vi "Engine 2 UI.vi"() -> ()   [LabVIEW 2015]
panel:
  out "Boolean_in":bool caption="Boolean"
  out "dbl_in":dbl caption="Double"
  out "String_in":string caption="String"
  out "U8_array_in":u8[](array[numeric]) caption="Array of U8"
  out "U8_in":u8 caption="U8"
  out "U16_in":u16 caption="U16"
  in  "Boolean_out":bool caption="Boolean"
  in  "dbl_out":dbl caption="Double"
  in  "String_out":string caption="String"
  in  "U8_array_out":u8[](array[numeric]) caption="Array of U8"
  in  "U8_out":u8 caption="U8"
  in  "U16_out":u16 caption="U16"
  out "Last Update":dbl format="%<%H:%M:%S>T"
  # "Input"
  # "Output"
  # "The UDP transfer mechanism allows the\nuser to configure a last update tag."
  # "Some data types are only compatible with\nspecific transfer mechanisms. For example:\nthe UDP transfer mechanism supports \nstrings and arrays, while the RT FIFO\ntransfer mechanism does not."
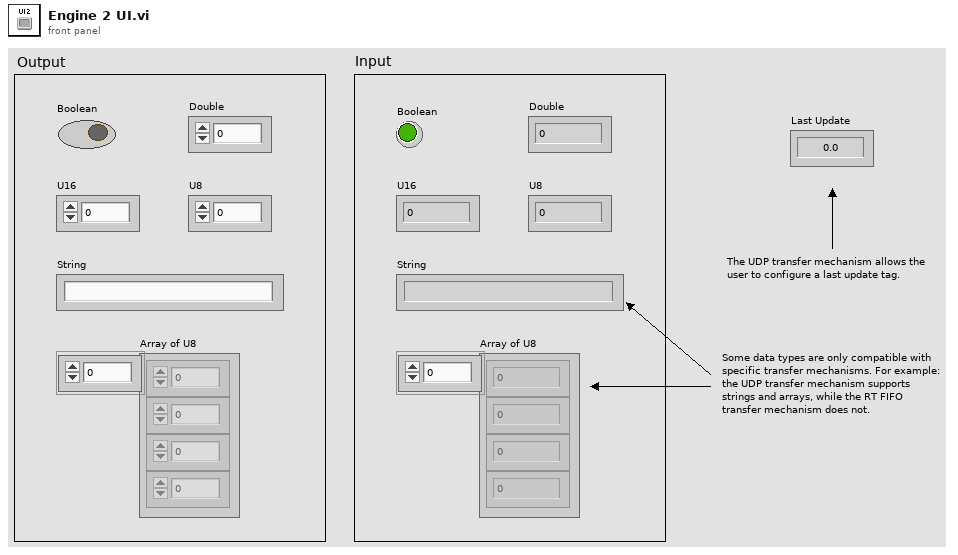
[diagram p1: front panel]
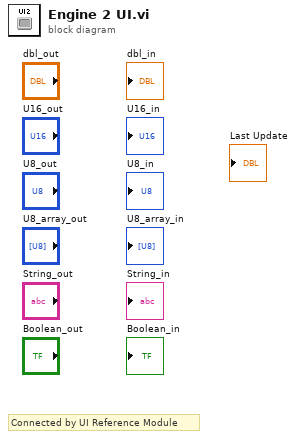
[diagram p0: block diagram]
diagram:
  # "Connected by UI Reference Module"
